vi "Get_Symbol_Index.vi"(8 "error in (no error)":errorcluster, 11 "IB_TreeItem in":refnum<class "IB_Tree_Item_Source_DotNET.lvclass">) -> (0 "error out":errorcluster, 2 "symbol index":i32, 3 "IB_TreeItem out":refnum<class "IB_Tree_Item_Source_DotNET.lvclass">)   [LabVIEW 2020, in "IB_Tree_Item_Source_DotNET.lvclass"]
uses:
  <vilib>/AppBuilder/IB_Classes/Tree_Item_Source_NET/IB_Tree_Item_Source_DotNET.lvclass
  <vilib>/AppBuilder/IB_Classes/Tree_Item_Source_NET/IB_Tree_Item_Source_DotNET.lvclass/IB_Tree_Item_Source_DotNET.ctl
  <resource>/Framework/Providers/Builds/Installer/controls/IB_Tree_DefaultSymbols.ctl
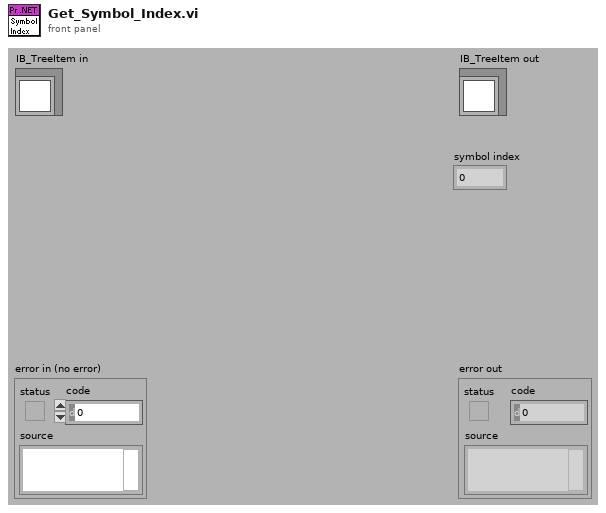
[diagram p1: front panel]
types:
  T1 = typedef "IB_Tree_DefaultSymbols.ctl" = enum16{"<unknown>", "closed folder", "open folder", "closed folder (default)", "open folder (default)", "closed sync folder", "open sync folder", "container folder", "my computer", "build specs", "exe", "dll", "source dist", "restful web service", ".net", "packed library", "c-generator", "target"}
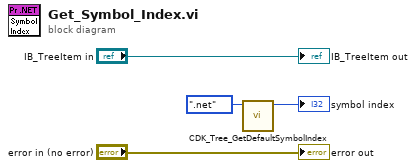
[diagram p0: block diagram]
diagram:
  n1 = call <resource>:"CDK_Tree_GetDefaultSymbolIndex.vi"("default symbol"=IB_Tree_DefaultSymbols.".net") -> ("symbol index"=→"symbol index":i32)  [unwired: 1 in, 9 out]
  "error out" <- "error in (no error)"
  "IB_TreeItem out" <- "IB_TreeItem in"
